vi "Write Library_Version to VIPB.vi"(8 "error in":errorcluster, 9 "Library_Version":string, 10 "VIPB File Path":path) -> (0 "error out":errorcluster)   [LabVIEW 2019, in "VIPM.lvlib"]
uses:
  VIPM.lvlib
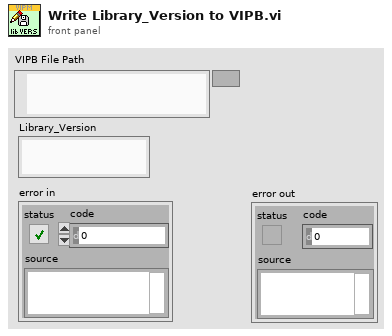
[diagram p1: front panel]
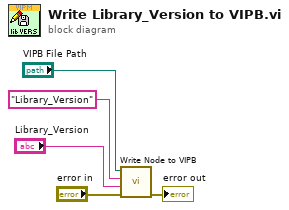
[diagram p0: block diagram]
diagram:
  n1 = call "Write Node to VIPB.vi"("error in (no error)"="error in", "New Text"="Library_Version", "Node Name"="Library_Version" ("XPath expression"), "VIPB File Path"="VIPB File Path") -> ("error out"=→"error out":errorcluster)  [unwired: 6 in, 1 out]
